vi "mp_sound_rt.vi"() -> ()   [LabVIEW 2023]
uses:
  <vilib>/sound2/lvsound2.llb/Sampling Mode.ctl
  <vilib>/sound2/lvsound2.llb/Sound Data Format.ctl
  <vilib>/sound2/lvsound2.llb/Sound File Write Open.vi
  <vilib>/sound2/lvsound2.llb/Sound Input Read (DBL).vi
  <vilib>/measure/maspectr.llb/FFT Spectrum (Mag-Phase) for N Chan.vi
  <vilib>/sound2/lvsound2.llb/Sound File Write (DBL).vi
  <vilib>/measure/NI_MAPro.lvlib
panel:
  out "phases":cluster{"f0":dbl, "df":dbl, "phase":dbl[]}[](graph)
  out "magnitudes'":cluster{"f0":dbl, "df":dbl, "magnitude":dbl[]}[](graph)
  in  "base path":path
  in  "file name":string
  out "appended path":path
  in  "number of samples/ch 2":i32=10000
  in  "device ID 2":u32
  out "Waveform Graph":waveform(dbl)[](graph)
  in  "Stop Button":bool
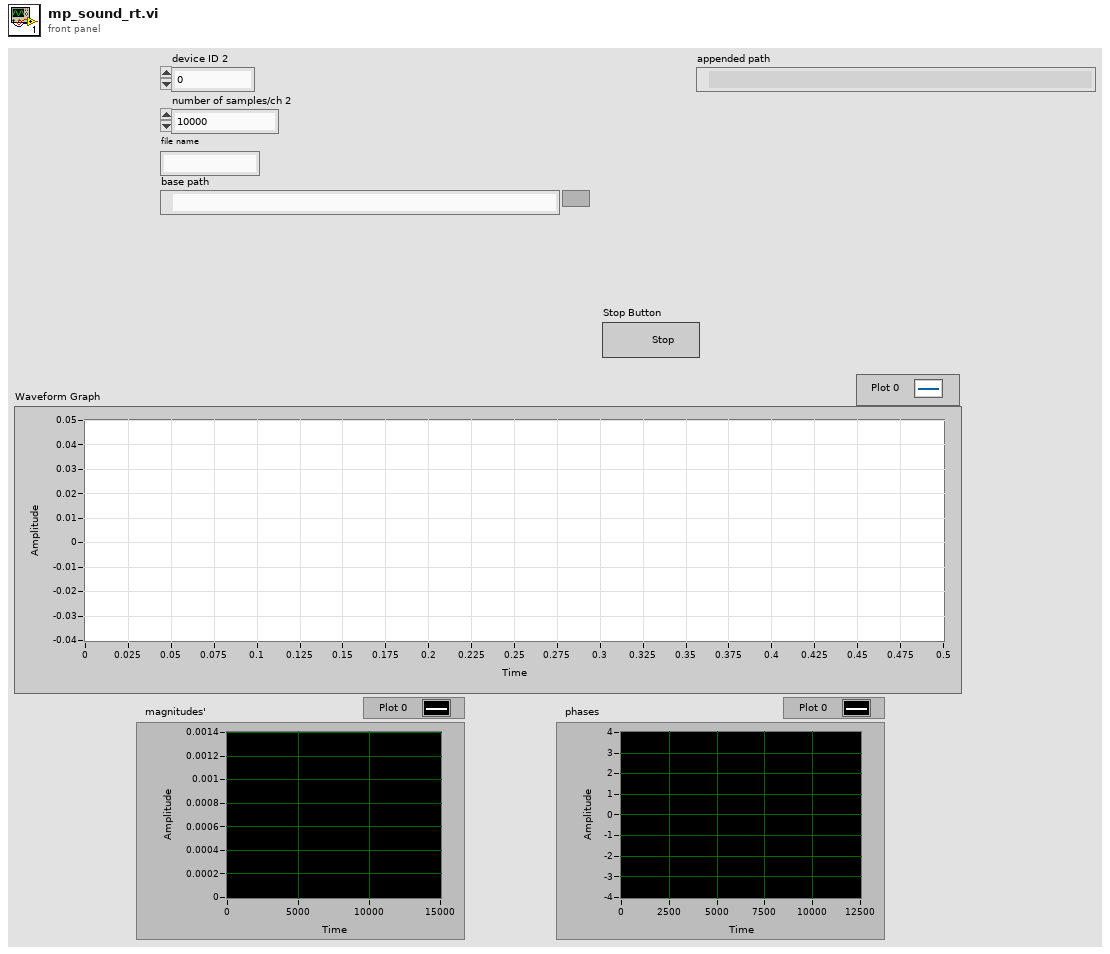
[diagram p1: front panel]
types:
  T1 = typedef "Sound Data Format.ctl" = cluster{"sample rate (S/s)":dbl, "number of channels":i32, "bits per sample":i32}
  T2 = typedef "Sampling Mode.ctl" = i32
  T3 = typedef "Sound File Refnum.ctl" = refnum<file>
  T4 = typedef "Sound Input Task ID.ctl" = u32
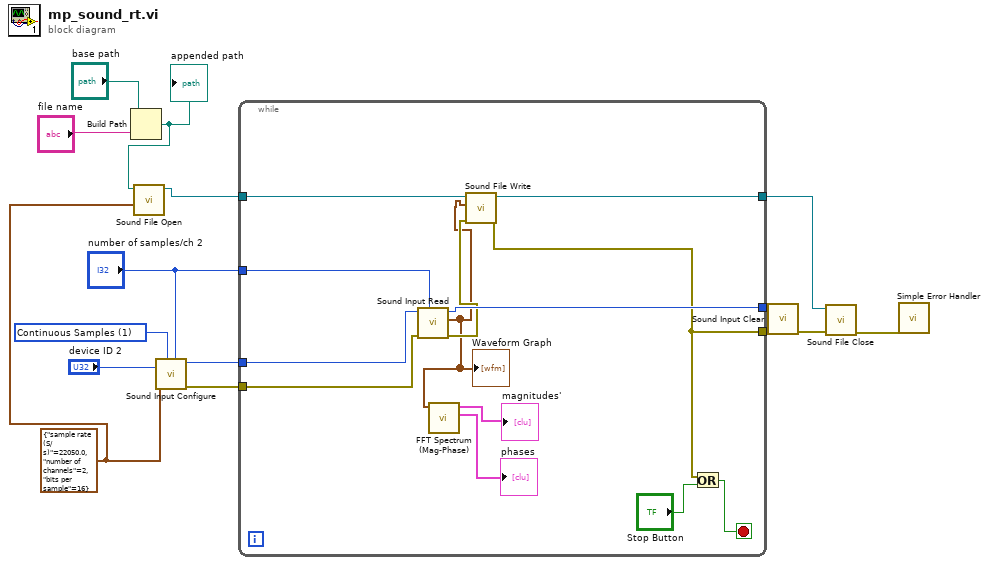
[diagram p0: block diagram]
diagram:
  w9 = T1 {"sample rate (S/s)"=22050.0, "number of channels"=2, "bits per sample"=16} ("sound format")
  w14 = T2 1 items=["Finite Samples", "Continuous Samples"] ("sample mode")
  n1 = Build Path(base path="base path", name or relative path="file name") -> (appended path=w8:path)
  "appended path" <- w8
  n2 = call-poly <vilib>:"Sound File Open.vi"("sound format"=w9, "path"=w8) -> ("sound file refnum"=w7:T3)  [unwired: 8 in, 1 out]
  n3 = call <vilib>:"Sound Input Configure.vi"("number of samples/ch"="number of samples/ch 2", "sample mode"=w14, "sound format"=w9, "device ID"="device ID 2") -> ("error out"=w11:errorcluster, "task ID"=w12:T4)  [unwired: 6 in]
  n4 = while {
    tunnel: "number of samples/ch 2" -> [w28]
    tunnel: w12 -> [w27]
    tunnel: w11 -> [w26]
    tunnel: [w25] -> w10
    tunnel: w7 -> [w22]
    tunnel: [w20] -> w6
    tunnel: [w19] -> w4
    stop <- w23 stop-if-true
    n5 = call-poly <vilib>:"Sound Input Read.vi"("number of samples/ch"=w28, "error in (no error)"=w26, "task ID"=w27) -> ("error out"=w21:errorcluster, "data"=w18:waveform(dbl)[], "task ID out"=w25:T4)  [unwired: 6 in]
    "Waveform Graph" <- w18
    n6 = call-poly <vilib>:"FFT Spectrum (Mag-Phase).vi"("time signals"=w18) -> ("phases"=→"phases":cluster{"f0":dbl, "df":dbl, "phase":dbl[]}[], "magnitudes"=→"magnitudes'":cluster{"f0":dbl, "df":dbl, "magnitude":dbl[]}[])  [unwired: 6 in, 3 out]
    n7 = call-poly <vilib>:"Sound File Write.vi"("error in (no error)"=w21, "data"=w18, "sound file refnum"=w22) -> ("error out"=w20:errorcluster, "sound file refnum out"=w19:T3)  [unwired: 7 in]
    n8 = Or(x=w20, y="Stop Button") -> (x .or. y?=w23:bool)
  }
  n9 = call <vilib>:"Sound Input Clear.vi"("error in (no error)"=w6, "task ID"=w10) -> ("error out"=w5:errorcluster)  [unwired: 9 in]
  n10 = call <vilib>:"Sound File Close.vi"("error in (no error)"=w5, "sound file refnum"=w4) -> ("error out"=w3:errorcluster)  [unwired: 9 in]
  n11 = call <vilib>:"Simple Error Handler.vi"("error in (no error)"=w3) -> ()  [unwired: 4 in, 5 out]
